vi "Read.vi"(8 "error in (no error)":errorcluster, 9 "Variant":variant, 11 "RS232 in":refnum<class "RS-xxx.lvclass">) -> (0 "error out":errorcluster, 2 "String":string, 3 "RS232 out":refnum<class "RS-xxx.lvclass">)   [LabVIEW 2023, in "Protocols.lvlib" / "RS-xxx.lvclass"]
uses:
  RS-xxx.lvclass
  Protocol Parent/Methods/Read Parameter.ctl
  Protocol Parent/Protocol Parent.lvclass
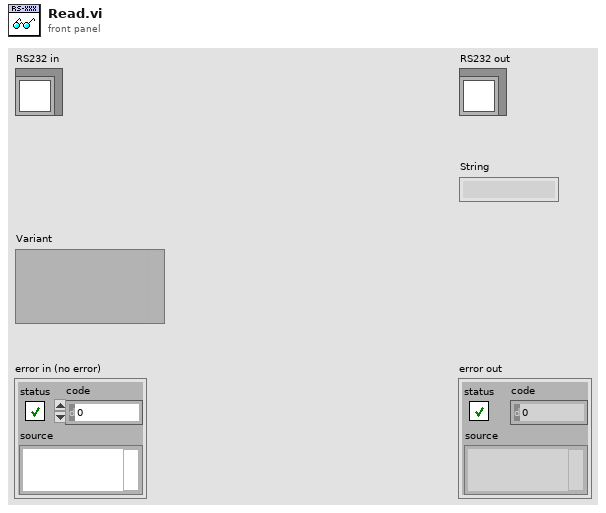
[diagram p1: front panel]
types:
  T1 = typedef "Protocols.lvlib/Protocol Parent.lvclass/Read Parameter.ctl" = cluster{"Wait Type":enum16{"Byte Count", "Wait sec"}, "Wait Value":dbl}
  T2 = cluster{"Port":string, "Baud Rate":u32, "Data Bits":u16, "Parity":enum16{"None", "Odd", "Even", "Mark", "Space"}, "Stop Bits":u16, "Flow Control":u16, "XON":enum16{"NUL", "SOH", "STX", "ETX", "EOT", "ENQ", "ACK", "BEL", "BS", "HT", "LF", "VT", "FF", "CR", "SO", "SI", "DLE", "DC1", "DC2", "DC3", "DC4", "NAK", "SYN", "ETB", "CAN", "EM", "SUB", "ESC", "FS", "GS", "RS", "US", "SP", "!", "\"", "#", "$", "%", "&", "'", "(", ")", "*", "+", ",", "- (-)", ".", "/", "0", "1", "2", "3", "4", "5", "6", "7", "8", "9", ":", ";", "<", "=", ">", "?", "@", "A", "B", "C", "D", "E", "F", "G", "H", "I", "J", "K", "L", "M", "N", "O", "P", "Q", "R", "S", "T", "U", "V", "W", "X", "Y", "Z", "[", "\\", "]", "^", "_", "`", "a", "b", "c", "d", "e", "f", "g", "h", "i", "j", "k", "l", "m", "n", "o", "p", "q", "r", "s", "t", "u", "v", "w", "x", "y", "z", "{", "|", "}", "~"}, "XOFF":enum16{"NUL", "SOH", "STX", "ETX", "EOT", "ENQ", "ACK", "BEL", "BS", "HT", "LF", "VT", "FF", "CR", "SO", "SI", "DLE", "DC1", "DC2", "DC3", "DC4", "NAK", "SYN", "ETB", "CAN", "EM", "SUB", "ESC", "FS", "GS", "RS", "US", "SP", "!", "\"", "#", "$", "%", "&", "'", "(", ")", "*", "+", ",", "- (-)", ".", "/", "0", "1", "2", "3", "4", "5", "6", "7", "8", "9", ":", ";", "<", "=", ">", "?", "@", "A", "B", "C", "D", "E", "F", "G", "H", "I", "J", "K", "L", "M", "N", "O", "P", "Q", "R", "S", "T", "U", "V", "W", "X", "Y", "Z", "[", "\\", "]", "^", "_", "`", "a", "b", "c", "d", "e", "f", "g", "h", "i", "j", "k", "l", "m", "n", "o", "p", "q", "r", "s", "t", "u", "v", "w", "x", "y", "z", "{", "|", "}", "~"}, "End Read on Termination Character":bool, "End Write on Termination Character":bool, "Termination Character":u8, "4wireMode":bool, "AssertDTR":bool, "WireMode":i16}
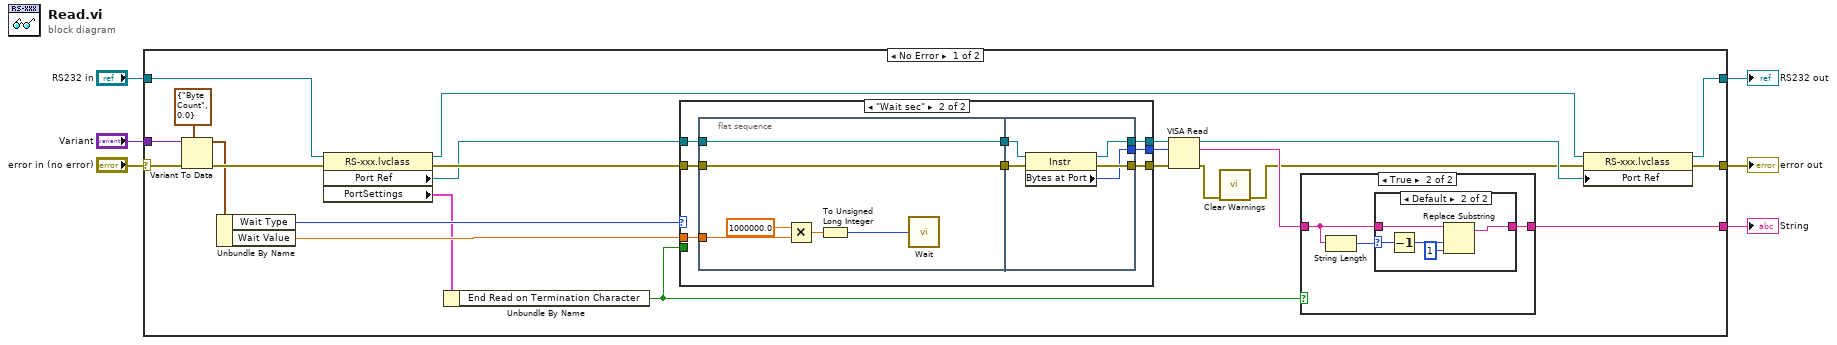
[diagram p0: block diagram]
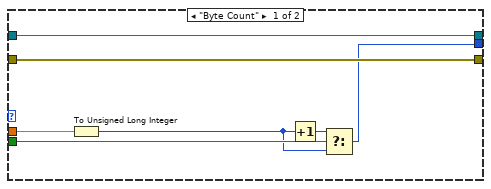
[diagram p4: hidden frame]
diagram:
  n1 = case shown="No Error" "error in (no error)" {
    selector: "error in (no error)" -> [w24 w67]
    tunnel: "RS232 in" -> [w29 w66]
    tunnel: [w27 w67] -> w2
    tunnel: [w25 w66] -> w4
    tunnel: "Variant" -> [w22 _]
    tunnel: [w10 _] -> w1
    frame No Error {
      n2 = Variant To Data(error in=w24, type=T1 {"Wait Type"=enum."Byte Count", "Wait Value"=0.0} ("Read Parameter"), Variant=w22) -> (data=w21:T1, error out=w23:errorcluster)
      n3 = Unbundle By Name(w21) -> ("Wait Type"=w15:enum16{"Byte Count", "Wait sec"}, "Wait Value"=w14:dbl)
      n4 = property class="RS-xxx.lvclass"(reference=w29, error in=w23) -> (reference out=w26:refnum<class "RS-xxx.lvclass">, error out=w20:errorcluster, "Port Ref"=w19:refnum<visa-resource-name>, "PortSettings"=w12:T2)
      n5 = Unbundle By Name(w12) -> ("End Read on Termination Character"=w9:bool)
      n6 = case shown="\"Wait sec\"" w15 {
        tunnel: w20 -> [w46 w54]
        tunnel: w19 -> [w45 w53]
        tunnel: [w46 w52] -> w18
        tunnel: [w45 w51] -> w17
        tunnel: [w41 w50] -> w16
        tunnel: w14 -> [w43 w47]
        tunnel: w9 -> [w44 _]
        frame "Byte Count" {
          n7 = To Unsigned Long Integer(number=w43) -> (unsigned 32bit integer=w40:u32)
          n8 = Increment(x=w40) -> (x+1=w42:u32)
          n9 = Select(t=w42, s=w44, f=w40) -> (s? t:f=w41:u32)
        }
        frame "Wait sec" {
          n10 = flat-sequence {
            tunnel: w53 -> [w59]
            tunnel: w54 -> [w60]
            tunnel: [w60] -> w49
            tunnel: [w59] -> w48
            tunnel: w47 -> [w56]
            tunnel: [w63] -> w52
            tunnel: [w62] -> w51
            tunnel: [w61] -> w50
            tunnel: w49 -> [w65]
            tunnel: w48 -> [w64]
            frame #0 {
              n11 = Multiply(x=1000000.0, y=w56) -> (x*y=w57:dbl)
              n12 = To Unsigned Long Integer(number=w57) -> (unsigned 32bit integer=w55:u32)
              n13 = call "Wait"("Count(uSec)"=w55) -> ()  [unwired: 1 out]
            }
            frame #1 {
              n14 = property class="Instr"(reference=w64, error in=w65) -> (reference out=w62:refnum<visa-resource-name>, error out=w63:errorcluster, "Bytes at Port"=w61:u32)
            }
          }
        }
      }
      n15 = VISA Read(VISA resource name=w17, byte count=w16, error in (no error)=w18) -> (VISA resource name out=w28:refnum<visa-resource-name>, read buffer=w11:string, error out=w8:errorcluster)  [unwired: 1 out]
      n16 = call "Clear Warnings.vi"("error in (no error)"=w8) -> ("error out"=w7:errorcluster)  [unwired: 10 in]
      n17 = case shown="True" w9 {
        tunnel: w11 -> [w30 w32]
        tunnel: [w30 w31] -> w10
        frame False {
        }
        frame True {
          n18 = String Length(string=w32) -> (length=w33:i32)
          n19 = case shown="Default" w33 {
            selector: w33 -> [_ w39]
            tunnel: w32 -> [w34 w37]
            tunnel: [w34 w36] -> w31
            frame 0 {
            }
            frame Default {
              n20 = Decrement(x=w39) -> (x-1=w38:i32)
              n21 = Replace Substring(2:1 ("length (len. of substring)"), 3:w38, 5:w37) -> (1:w36:string)  [unwired: 1 in, 1 out]
            }
          }
        }
      }
      n22 = property class="RS-xxx.lvclass"(reference=w26, error in=w7, "Port Ref"=w28) -> (reference out=w25:refnum<class "RS-xxx.lvclass">, error out=w27:errorcluster)
    }
    frame Error {
    }
  }
  "error out" <- w2
  "RS232 out" <- w4
  "String" <- w1
